vi "BarLIV_SearchAndPlot_Main.vi"() -> ()   [LabVIEW 2017]
uses:
  <vilib>/Utility/NIReport.llb/NI_report.lvclass
panel:
  out "Data Selected (<10)":string[][](array[string])
  in  "Stop and Plot":bool
  in  "Input File Name":string="report_1"
  in  "File Directory to Save Report":path=path "D:/LabVIEW_prog/Trumpf_Database_Connect/Report_output"
  in  "Excel Template":path=path "D:/LabVIEW_prog/Trumpf_Database_Connect/Bar_LIV_ExcelTemp.xlsx"
  out "Select Data":string[][](array[string])=[["23", "3/22/2019", "30101566", "DM17-20                  ", "                         ", "Fail", "30", "0.14", "1.375", "934.203", "37.774", "0.339"], ["24", "3/22/2019", "30101566", "DM17-20                  ", "                         ", "Fail", "60", "25.11", "1.413", "935.39", "41.68", "29.618"], ["25", "3/22/2019", "30101566", "DM17-20                  ", "                         ", "Fail", "90", "58.98", "1.444", "936.11", "44.048", "45.383"], ["26", "3/22/2019", "30101566", "DM17-20                  ", "                         ", "Fail", "120", "93.3", "1.473", "936.93", "46.745", "52.783"], ["27", "3/22/2019", "30101566", "DM17-20                  ", "                         ", "Fail", "150", "127.7", "1.502", "937.91", "49.969", "56.68"], ["28", "3/22/2019", "30101566", "DM17-20                  ", "                         ", "Fail", "180", "161.8", "1.53", "938.84", "53.028", "58.751"], ["29", "3/22/2019", "30101566", "DM17-20                  ", "                         ", "Fail", "210", "195.3", "1.558", "939.97", "56.745", "59.692"], ["30", "3/22/2019", "30101566", "DM17-20                  ", "                         ", "Fail", "240", "228.2", "1.584", "941.04", "60.265", "60.027"], ["31", "3/22/2019", "30101566", "DM17-20                  ", "                         ", "Fail", "270", "260.1", "1.61", "942.37", "64.64", "59.834"], ["32", "3/22/2019", "30101566", "DM17-20                  ", "                         ", "Fail", "300", "290.9", "1.635", "943.75", "69.18", "59.307"], ["33", "3/22/2019", "30101566", "DM17-20                  ", "                         ", "Fail", "330", "320.2", "1.66", "945.28", "74.212", "58.452"]]
  out "Raw Bar Table Data":string[][](array[string])=[["1", "3/22/2019", "30101152", "DM17-20                  ", "                         ", "31 emitters/Pass", "30", "0.06", "1.375", "933.884", "37.774", "0.145"], ["2", "3/22/2019", "30101152", "DM17-20                  ", "                         ", "31 emitters/Pass", "60", "24.48", "1.414", "935.13", "41.871", "28.854"], ["3", "3/22/2019", "30101152", "DM17-20                  ", "                         ", "31 emitters/Pass", "90", "57.61", "1.445", "935.9", "44.404", "44.298"], ["4", "3/22/2019", "30101152", "DM17-20                  ", "                         ", "31 emitters/Pass", "120", "91.3", "1.475", "936.78", "47.298", "51.582"], ["5", "3/22/2019", "30101152", "DM17-20                  ", "                         ", "31 emitters/Pass", "150", "125", "1.504", "937.76", "50.522", "55.408"], ["6", "3/22/2019", "30101152", "DM17-20                  ", "                         ", "31 emitters/Pass", "180", "158.3", "1.532", "938.84", "54.075", "57.405"], ["7", "3/22/2019", "30101152", "DM17-20                  ", "                         ", "31 emitters/Pass", "210", "191.3", "1.56", "939.97", "57.792", "58.394"], ["8", "3/22/2019", "30101152", "DM17-20                  ", "                         ", "31 emitters/Pass", "240", "222.8", "1.587", "941.25", "62.002", "58.496"], ["9", "3/22/2019", "30101152", "DM17-20                  ", "                         ", "31 emitters/Pass", "270", "253.6", "1.613", "942.63", "66.542", "58.231"], ["10", "3/22/2019", "30101152", "DM17-20                  ", "                         ", "31 emitters/Pass", "300", "282.9", "1.639", "944.11", "71.41", "57.535"], ["11", "3/22/2019", "30101152", "DM17-20                  ", "                         ", "31 emitters/Pass", "330", "311.2", "1.664", "945.73", "76.739", "56.672"], ["12", "3/22/2019", "30101562", "DM17-20                  ", "                         ", "Pass", "30", "0.18", "1.374", "934.413", "37.888", "0.437"], ["13", "3/22/2019", "30101562", "DM17-20                  ", "                         ", "Pass", "60", "25.92", "1.413", "935.59", "41.76", "30.573"], ["14", "3/22/2019", "30101562", "DM17-20                  ", "                         ", "Pass", "90", "59.94", "1.443", "936.37", "44.326", "46.154"], ["15", "3/22/2019", "30101562", "DM17-20                  ", "                         ", "Pass", "120", "94.3", "1.473", "937.19", "47.023", "53.349"], ["16", "3/22/2019", "30101562", "DM17-20                  ", "                         ", "Pass", "150", "128.7", "1.502", "938.12", "50.083", "57.124"], ["17", "3/22/2019", "30101562", "DM17-20                  ", "                         ", "Pass", "180", "162.8", "1.53", "939.14", "53.438", "59.114"], ["18", "3/22/2019", "30101562", "DM17-20                  ", "                         ", "Pass", "210", "196.5", "1.557", "940.27", "57.155", "60.097"], ["19", "3/22/2019", "30101562", "DM17-20                  ", "                         ", "Pass", "240", "229.2", "1.584", "941.5", "61.201", "60.29"], ["20", "3/22/2019", "30101562", "DM17-20                  ", "                         ", "Pass", "270", "261", "1.61", "942.83", "65.576", "60.041"], ["21", "3/22/2019", "30101562", "DM17-20                  ", "                         ", "Pass", "300", "291.7", "1.635", "944.21", "70.115", "59.47"], ["22", "3/22/2019", "30101562", "DM17-20                  ", "                         ", "Pass", "330", "320.8", "1.659", "945.83", "75.444", "58.597"], ["23", "3/22/2019", "30101566", "DM17-20                  ", "                         ", "Fail", "30", "0.14", "1.375", "934.203", "37.774", "0.339"], ["24", "3/22/2019", "30101566", "DM17-20                  ", "                         ", "Fail", "60", "25.11", "1.413", "935.39", "41.68", "29.618"], ["25", "3/22/2019", "30101566", "DM17-20                  ", "                         ", "Fail", "90", "58.98", "1.444", "936.11", "44.048", "45.383"], ["26", "3/22/2019", "30101566", "DM17-20                  ", "                         ", "Fail", "120", "93.3", "1.473", "936.93", "46.745", "52.783"], ["27", "3/22/2019", "30101566", "DM17-20                  ", "                         ", "Fail", "150", "127.7", "1.502", "937.91", "49.969", "56.68"], ["28", "3/22/2019", "30101566", "DM17-20                  ", "                         ", "Fail", "180", "161.8", "1.53", "938.84", "53.028", "58.751"], ["29", "3/22/2019", "30101566", "DM17-20                  ", "                         ", "Fail", "210", "195.3", "1.558", "939.97", "56.745", "59.692"], ["30", "3/22/2019", "30101566", "DM17-20                  ", "                         ", "Fail", "240", "228.2", "1.584", "941.04", "60.265", "60.027"], ["31", "3/22/2019", "30101566", "DM17-20                  ", "                         ", "Fail", "270", "260.1", "1.61", "942.37", "64.64", "59.834"], ["32", "3/22/2019", "30101566", "DM17-20                  ", "                         ", "Fail", "300", "290.9", "1.635", "943.75", "69.18", "59.307"], ["33", "3/22/2019", "30101566", "DM17-20                  ", "                         ", "Fail", "330", "320.2", "1.66", "945.28", "74.212", "58.452"], ["34", "3/22/2019", "30101586", "DM17-20                  ", "                         ", "Pass", "30", "0.12", "1.375", "934.057", "37.55", "0.291"], ["35", "3/22/2019", "30101586", "DM17-20                  ", "                         ", "Pass", "60", "24.93", "1.415", "935.23", "41.41", "29.364"], ["36", "3/22/2019", "30101586", "DM17-20                  ", "                         ", "Pass", "90", "58.6", "1.447", "935.95", "43.778", "44.997"], ["37", "3/22/2019", "30101586", "DM17-20                  ", "                         ", "Pass", "120", "92.9", "1.478", "936.78", "46.509", "52.379"], ["38", "3/22/2019", "30101586", "DM17-20                  ", "                         ", "Pass", "150", "127.3", "1.507", "937.71", "49.568", "56.315"], ["39", "3/22/2019", "30101586", "DM17-20                  ", "                         ", "Pass", "180", "161.3", "1.537", "938.68", "52.759", "58.303"], ["40", "3/22/2019", "30101586", "DM17-20                  ", "                         ", "Pass", "210", "194.7", "1.565", "939.76", "56.311", "59.242"], ["41", "3/22/2019", "30101586", "DM17-20                  ", "                         ", "Pass", "240", "227.6", "1.593", "940.89", "60.028", "59.531"], ["42", "3/22/2019", "30101586", "DM17-20                  ", "                         ", "Pass", "270", "259.4", "1.62", "942.12", "64.075", "59.305"], ["43", "3/22/2019", "30101586", "DM17-20                  ", "                         ", "Pass", "300", "290.1", "1.647", "943.49", "68.581", "58.713"], ["44", "3/22/2019", "30101586", "DM17-20                  ", "                         ", "Pass", "330", "319.4", "1.673", "945.02", "73.614", "57.853"], ["45", "3/22/2019", "30101731", "DM17-20                  ", "                         ", "31 emitters/Pass", "30", "0.18", "1.375", "933.644", "37.885", "0.436"], ["46", "3/22/2019", "30101731", "DM17-20                  ", "                         ", "31 emitters/Pass", "60", "24.92", "1.415", "934.87", "41.92", "29.352"], ["47", "3/22/2019", "30101731", "DM17-20                  ", "                         ", "31 emitters/Pass", "90", "58.52", "1.446", "935.64", "44.453", "44.967"], ["48", "3/22/2019", "30101731", "DM17-20                  ", "                         ", "31 emitters/Pass", "120", "92.7", "1.475", "936.47", "47.183", "52.373"], ["49", "3/22/2019", "30101731", "DM17-20                  ", "                         ", "31 emitters/Pass", "150", "126.8", "1.505", "937.45", "50.407", "56.168"], ["50", "3/22/2019", "30101731", "DM17-20                  ", "                         ", "31 emitters/Pass", "180", "160.3", "1.533", "938.48", "53.795", "58.092"], ["51", "3/22/2019", "30101731", "DM17-20                  ", "                         ", "31 emitters/Pass", "210", "192.9", "1.561", "939.55", "57.314", "58.845"], ["52", "3/22/2019", "30101731", "DM17-20                  ", "                         ", "31 emitters/Pass", "240", "224.9", "1.588", "940.73", "61.196", "59.01"], ["53", "3/22/2019", "30101731", "DM17-20                  ", "                         ", "31 emitters/Pass", "270", "255.6", "1.614", "942.06", "65.571", "58.653"], ["54", "3/22/2019", "30101731", "DM17-20                  ", "                         ", "31 emitters/Pass", "300", "285.6", "1.64", "943.54", "70.439", "58.049"], ["55", "3/22/2019", "30101731", "DM17-20                  ", "                         ", "31 emitters/Pass", "330", "313.9", "1.665", "945.12", "75.637", "57.13"]]
  in  "Finish Selection":bool
  out "Error Out":errorcluster
  in  "Error In":errorcluster
  in  "Wafer ID":string(combo)
  in  "Bar Work Order":string(combo)="DM17-20                  "
  in  "Bar Serial Num":string(combo)="30101566"
  in  "Test Date":string(combo)="3/22/2019"
  # "Bar LIV Selection From RD Database - Chao Gong"
  # "Note: \n1) Select test date, bar SN, work order, and wafer ID. (Leave it blank for all selection). \n2) Click finish selection.\n3) Click stop to save excel file and generate plotting report\n4) No more 10 selection a time (Excel template runs out)"
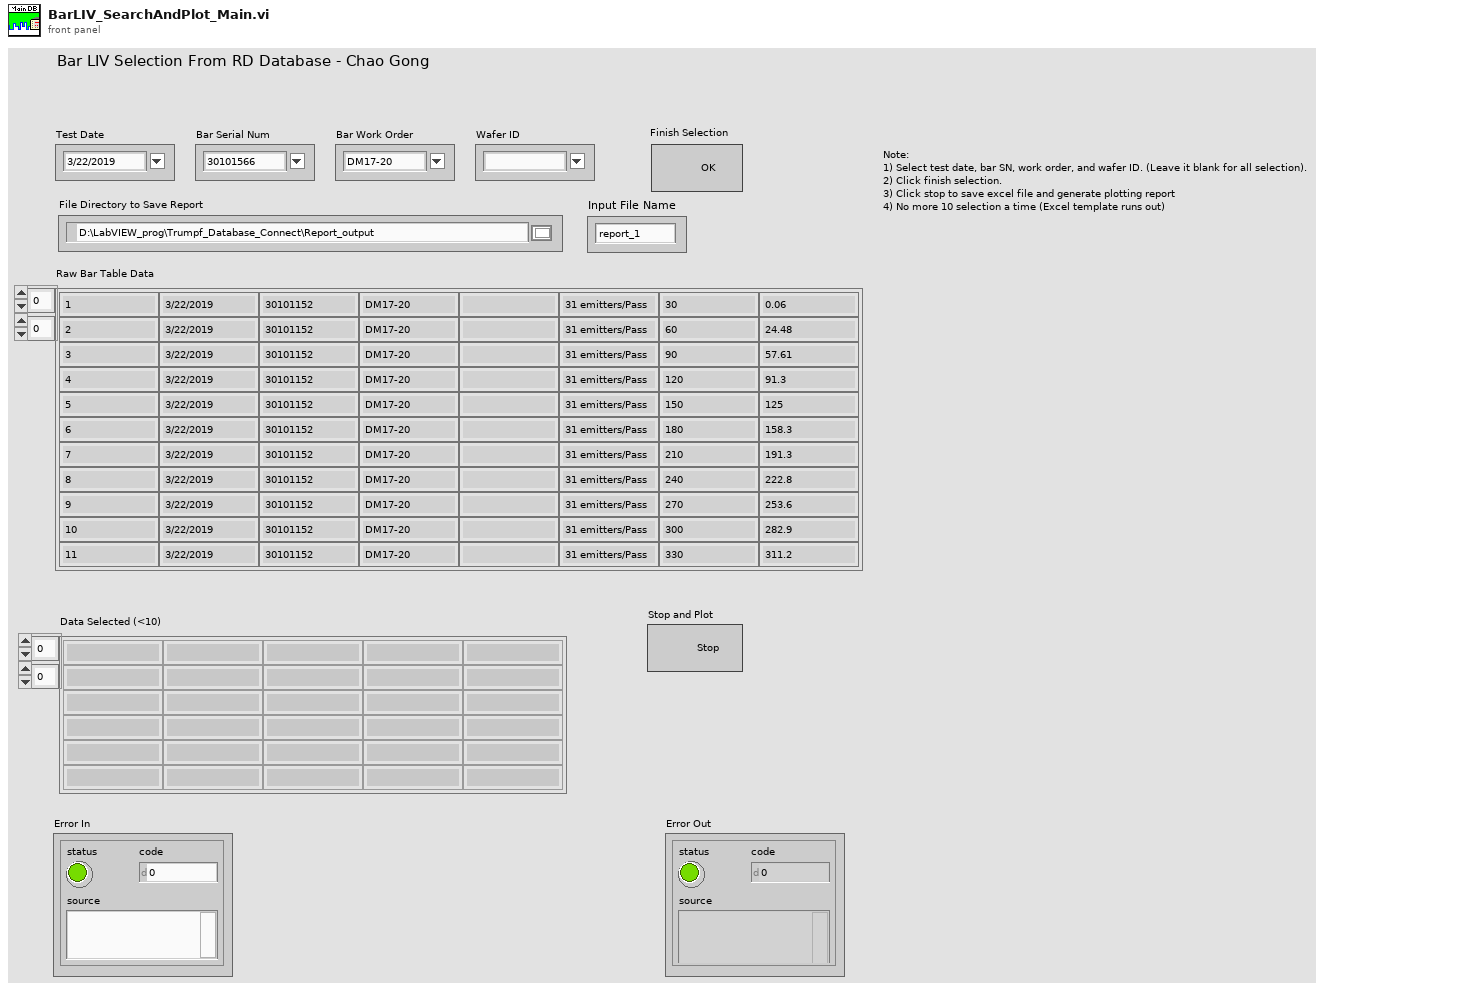
[diagram p1: front panel]
types:
  T1 = enum16{"Standard Report", "HTML", "Word", "Excel"}
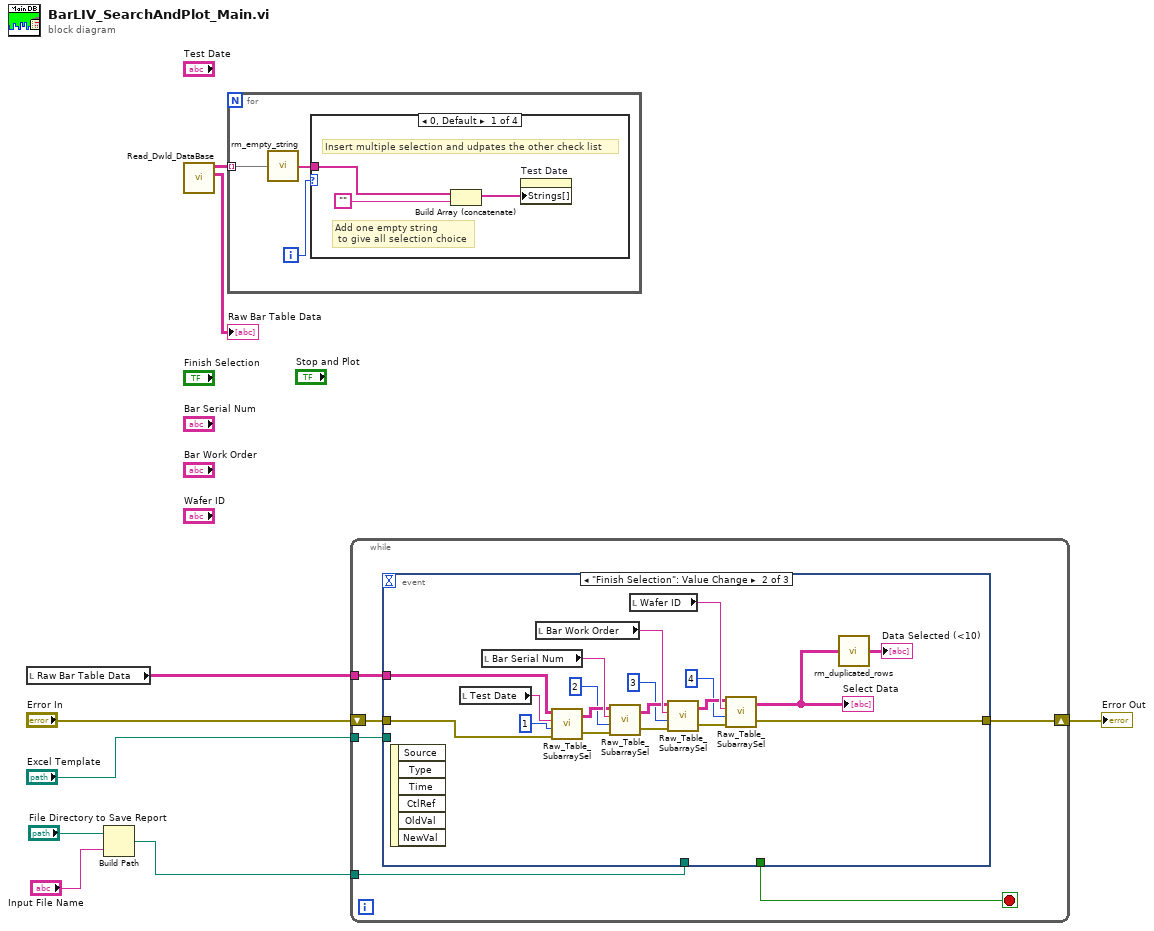
[diagram p0: block diagram]
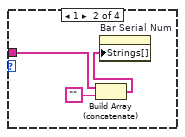
[diagram p2: hidden frame]
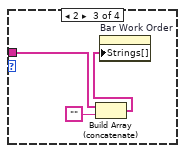
[diagram p3: hidden frame]
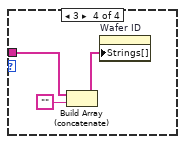
[diagram p4: hidden frame]
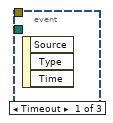
[diagram p5: hidden frame]
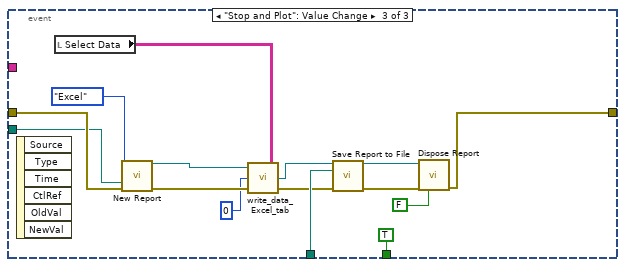
[diagram p6: hidden frame]
diagram:
  n1 = local read "Raw Bar Table Data"() -> (w7:string[][])
  n2 = Build Path(base path="File Directory to Save Report", name or relative path="Input File Name") -> (appended path=w2:path)
  n3 = call "Read_Dwld_DataBase.vi"() -> ("Output Data"=→"Raw Bar Table Data":string[][], "Output selection string"=w9:string[][])  [unwired: 4 in, 2 out]
  n4 = for {
    tunnel: w9 -> [w11] mode=indexing
    i -> [w12]
    n5 = call "rm_empty_string.vi"("Array"=w11) -> ("String output"=w10:string[])
    n6 = case shown="0, Default" w12 {
      tunnel: w10 -> [w14 w17 w20 w23]
      frame 0, Default {
        # "Insert multiple selection and udpates the other check list"
        # "Add one empty string\n to give all selection choice"
        n7 = Build Array (concatenate)(w14, "") -> (w13:string[])
        n8 = property on="Test Date" class="CmbBox"("Strings[]"=w13) -> ()  [unwired: 2 in, 2 out]
      }
      frame 1 {
        n9 = Build Array (concatenate)(w17, "") -> (w16:string[])
        n10 = property on="Bar Serial Num" class="CmbBox"("Strings[]"=w16) -> ()  [unwired: 2 in, 2 out]
      }
      frame 2 {
        n11 = Build Array (concatenate)(w20, "") -> (w19:string[])
        n12 = property on="Bar Work Order" class="CmbBox"("Strings[]"=w19) -> ()  [unwired: 2 in, 2 out]
      }
      frame 3 {
        n13 = Build Array (concatenate)(w23, "") -> (w22:string[])
        n14 = property on="Wafer ID" class="CmbBox"("Strings[]"=w22) -> ()  [unwired: 2 in, 2 out]
      }
    }
  }
  n15 = while {
    tunnel: w7 -> [w30]
    shift-right: [w28] -> w5
    shift-left: "Error In" -> [w29]
    tunnel: "Excel Template" -> [w27]
    tunnel: w2 -> [w26]
    stop <- w25 stop-if-true
    n16 = event shown="[1] \"Finish Selection\": Value Change" {
      selector: _ -> [_ _ _]
      dyn-events: _ -> [_ _ _]
      timeout: _ -> [_ _ _]
      tunnel: w30 -> [_ w33 _]
      tunnel: w29 -> [_ w38 w62]
      tunnel: [_ w34 w57] -> w28
      tunnel: w27 -> [_ _ w60]
      tunnel: w26 -> [_ _ w54]
      tunnel: [_ _ TRUE ("Stop Search and Plot")] -> w25
      event Timeout {
        n17 = event-data() -> ()  [unwired: 1 in, 3 out]
      }
      event "Finish Selection": Value Change {
        n18 = event-data() -> ()  [unwired: 1 in, 6 out]
        n19 = local read "Test Date"() -> (w49:string)
        n20 = local read "Bar Serial Num"() -> (w47:string)
        n21 = local read "Bar Work Order"() -> (w44:string)
        n22 = call "Raw_Table_SubarraySel.vi"("error in (no error)"=w38, "Column Index"=1, "String to compare"=w49, "Raw Bar Table Data"=w33) -> ("error out"=w37:errorcluster, "Output"=w46:string[][])
        n23 = call "Raw_Table_SubarraySel.vi"("error in (no error)"=w37, "Column Index"=2, "String to compare"=w47, "Raw Bar Table Data"=w46) -> ("error out"=w36:errorcluster, "Output"=w43:string[][])
        n24 = local read "Wafer ID"() -> (w41:string)
        n25 = call "Raw_Table_SubarraySel.vi"("error in (no error)"=w36, "Column Index"=3, "String to compare"=w44, "Raw Bar Table Data"=w43) -> ("error out"=w35:errorcluster, "Output"=w40:string[][])
        n26 = call "Raw_Table_SubarraySel.vi"("error in (no error)"=w35, "Column Index"=4, "String to compare"=w41, "Raw Bar Table Data"=w40) -> ("error out"=w34:errorcluster, "Output"=w32:string[][])
        "Select Data" <- w32
        n27 = call "rm_duplicated_rows.vi"("Select Data"=w32) -> ("Output Data"=→"Data Selected (<10)":string[][])
      }
      event "Stop and Plot": Value Change {
        n28 = event-data() -> ()  [unwired: 1 in, 6 out]
        n29 = local read "Select Data"() -> (w64:string[][])
        n30 = call <vilib>:"New Report.vi"("report type"=T1."Excel", "template (empty)"=w60, "error in (no error)"=w62) -> ("report out"=w63:refnum<class "NI_report.lvclass">, "error out"=w61:errorcluster)  [unwired: 3 in, 8 out]
        n31 = call "write_data_Excel_tab.vi"("text data"=w64, "error in (no error)"=w61, "worksheet index (0)"=0, "report in"=w63) -> ("error out"=w53:errorcluster, "report out"=w55:refnum<class "NI_report.lvclass">)
        n32 = call-dynamic "Save Report to File.vi"("report in"=w55, "report file path"=w54, "error in (no error)"=w53) -> ("report out"=w52:refnum<class "NI_report.lvclass">, "error out"=w51:errorcluster)  [unwired: 11 in]
        n33 = call-dynamic "Dispose Report.vi"("report in"=w52, "error in (no error)"=w51, "close report? (T)"=FALSE) -> ("error out"=w57:errorcluster)  [unwired: 12 in]
      }
    }
  }
  "Error Out" <- w5
